vi "Remove Correction Table Single Entry.vi"(8 "error in (no error)":errorcluster, 9 "Frequency (24MHz)":dbl=24000000.0 format="%#.9p", 10 "Correction Table (\"Table1\")":string="Table1", 11 "VISA resource name":refnum<visa-resource-name>) -> (0 "error out":errorcluster, 3 "VISA resource name out":refnum<visa-resource-name>)   [LabVIEW 2015, in "Rohde&Schwarz CMXP Base.lvlib"]
doc: "Removes a single entry from an existing correction table.\n\nAttribute:\n-\n\nRemote-control command:\nREMove:SYSTem:ATTenuation:CTABle"
uses:
  <instrlib>/Rohde&Schwarz CMXP Base/Rohde&Schwarz CMXP Base.lvlib
  <instrlib>/Rohde&Schwarz CMXP Base/Private/rsidr_core.llb/rsidr_core.lvlib
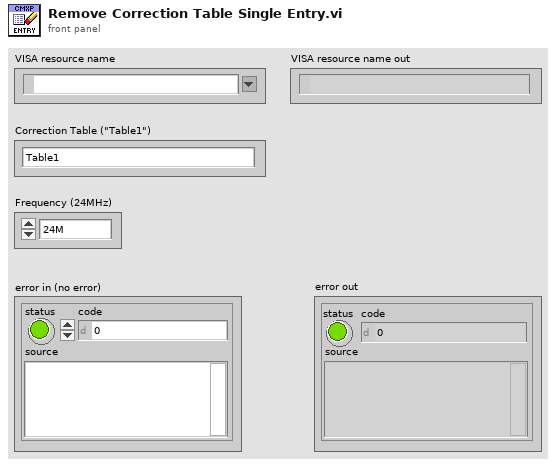
[diagram p1: front panel]
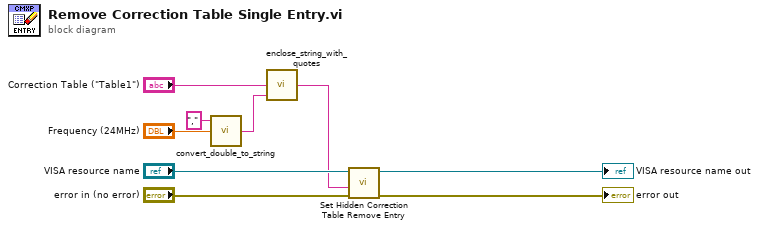
[diagram p0: block diagram]
diagram:
  n1 = call <instrlib>:"convert_double_to_string.vi"("double in"="Frequency (24MHz)", "String to add before (\"\")"="," ("String to add before (\"\")")) -> ("string out"=w2:string)  [unwired: 3 in]
  n2 = call <instrlib>:"enclose_string_with_quotes.vi"("String after"=w2, "String to enclose"="Correction Table (\"Table1\")") -> ("String out"=w1:string)  [unwired: 3 in]
  n3 = call "Set Hidden Correction Table Remove Entry"("error in (no error)"="error in (no error)", "Hidden Correction Table Remove Entry ()"=w1, "instrument handle"="VISA resource name") -> ("error out"=→"error out":errorcluster, "instrument handle out"=→"VISA resource name out":refnum<visa-resource-name>)  [unwired: 7 in]
